vi "DSF.Shared.Timing.Set Priority.vi"(10 "Priority":T1, 11 "Timing in":refnum<class "DSF.Shared.Timing.lvclass">) -> (3 "Timing out":refnum<class "DSF.Shared.Timing.lvclass">)   [LabVIEW 2017, in "DSF.Shared.lvlib" / "DSF.Shared.Timing.lvclass"]
uses:
  DSF.Shared.Timing.lvclass
  Typedefs/DSF.Shared.Typedefs.Scalars.Priority.ctl
  DSF.Shared.Timing.lvclass/DSF.Shared.Timing.ctl
  DSF.Shared.lvlib
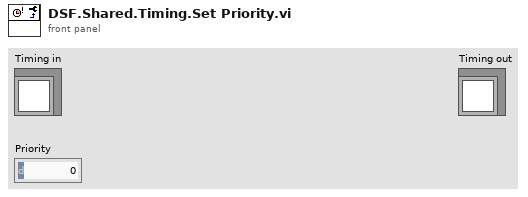
[diagram p1: front panel]
types:
  T1 = typedef "DSF.Shared.lvlib/DSF.Shared.Typedefs.Scalars.Priority.ctl" = u64
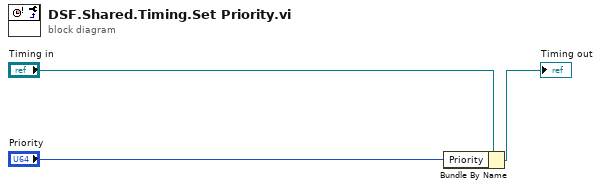
[diagram p0: block diagram]
diagram:
  n1 = Bundle By Name(cluster="Timing in", "Priority"="Priority") -> (→"Timing out":refnum<class "DSF.Shared.Timing.lvclass">)
